vi "Embed 2D to 3D.vi"(7 "Z":dbl, 8 "2D Point":T1) -> (2 "3D Point":T2)   [LabVIEW 2011]
uses:
  3D Point.ctl
  LIDAR Acquisition Loop/Simulation/2D Point.ctl
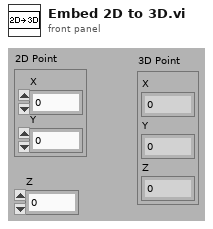
[diagram p1: front panel]
types:
  T1 = typedef "2D Point.ctl" = cluster{"X":dbl, "Y":dbl}
  T2 = typedef "3D Point.ctl" = cluster{"X":dbl, "Y":dbl, "Z":dbl}
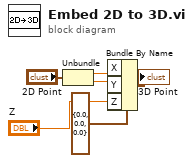
[diagram p0: block diagram]
diagram:
  n1 = Unbundle("2D Point") -> ("X"=w2:dbl, "Y"=w3:dbl)
  n2 = Bundle By Name(cluster=T2 {"X"=0.0, "Y"=0.0, "Z"=0.0} ("3D Point"), "X"=w2, "Y"=w3, "Z"="Z") -> (→"3D Point":T2)
